vi "start.vi"(8 "error in (no error)":errorcluster, 11 "FlukeDMM in":refnum<class "FlukeDMM.lvclass">) -> (0 "error out":errorcluster, 3 "FlukeDMM out":refnum<class "FlukeDMM.lvclass">)   [LabVIEW 2013, in "FlukeDMM.lvlib" / "FlukeDMM.lvclass"]
uses:
  <userlib>/Common/Devices/FlukeDMM/FlukeDMM/FlukeDMM.lvclass
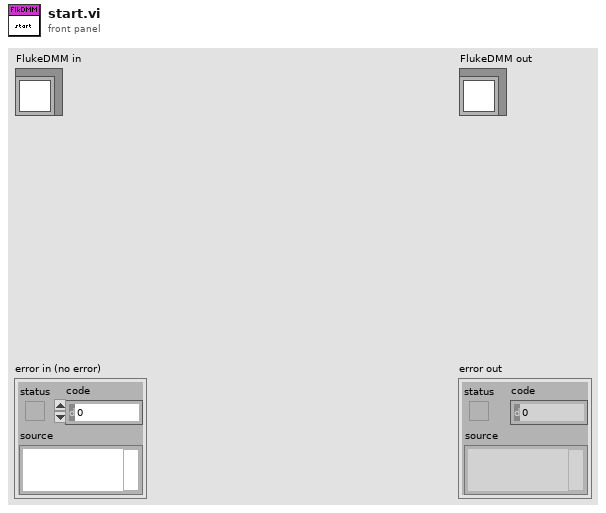
[diagram p1: front panel]
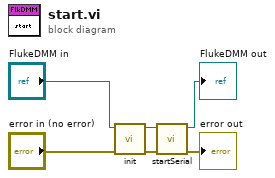
[diagram p0: block diagram]
diagram:
  n1 = call-dynamic "init.vi"("error in (no error)"="error in (no error)", "FlukeDMM in"="FlukeDMM in") -> ("error out"=w3:errorcluster, "FlukeDMM out"=w6:refnum<class "FlukeDMM.lvclass">)  [unwired: 8 in]
  n2 = call <userlib>:"startSerial.vi"("error in (no error)"=w3, "FlukeDMM in"=w6) -> ("error out"=→"error out":errorcluster, "FlukeDMM out"=→"FlukeDMM out":refnum<class "FlukeDMM.lvclass">)  [unwired: 8 in]
